vi "例4-21.vi"() -> ()   [LabVIEW 2019]
uses:
  <vilib>/Utility/file.llb/Read Delimited Spreadsheet (DBL).vi
panel:
  out "读出的数据":dbl[][](array[numeric]) format="%#_4g"
  in  "读数据列数":dbl=5.0
  in  "文件路径":path=path "d:/wave_sine.xls"
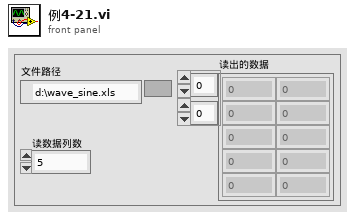
[diagram p1: front panel]
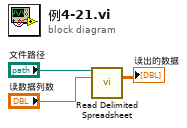
[diagram p0: block diagram]
diagram:
  n1 = call-poly <vilib>:"Read Delimited Spreadsheet.vi"("file path (dialog if empty)"="文件路径", "number of rows (all:-1)"="读数据列数") -> ("all rows"=→"读出的数据":dbl[][])  [unwired: 8 in, 5 out]
